vi "Get Module from Connection UI Element.vi"(10 "Alias or Full Endpoint":string, 11 "Alias Mappings by Module":T1[](array[typedef])) -> (1 "Long Endpoint":string, 2 "Short Endpoint":string, 3 "Module":string)   [LabVIEW 2020, in "Routing and Faulting System Explorer.lvlib"]
uses:
  Routing and Faulting System Explorer.lvlib
  Alias Map by Module.ctl
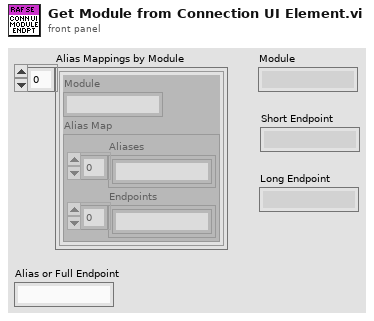
[diagram p1: front panel]
types:
  T1 = typedef "Routing and Faulting System Explorer.lvlib/Alias Map by Module.ctl" = cluster{"Module":string, "Alias Map":cluster{"Aliases":string[], "Endpoints":string[]}}
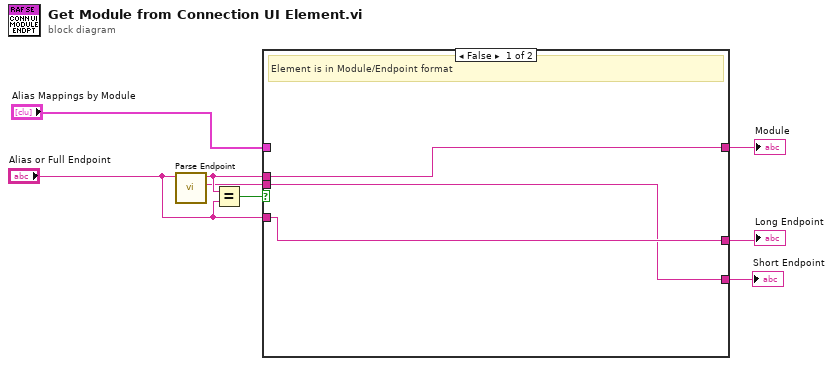
[diagram p0: block diagram]
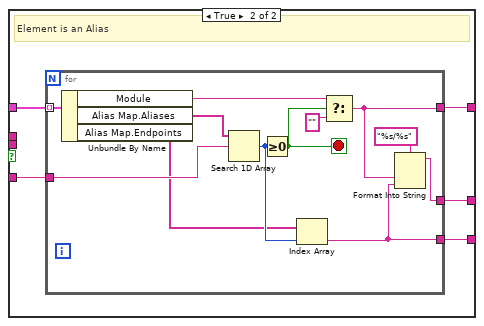
[diagram p2: hidden frame]
diagram:
  n1 = call "Parse Endpoint.vi"("Module/Endpoint"="Alias or Full Endpoint") -> ("Endpoint"=w4:string, "Module"=w6:string)  [unwired: 9 in]
  n2 = Equal?(x=w6, y="Alias or Full Endpoint") -> (x = y?=w5:bool)
  n3 = case shown="False" w5 {
    tunnel: "Alias Mappings by Module" -> [_ w16]
    tunnel: w6 -> [w11 _]
    tunnel: [w11 w15] -> w8
    tunnel: "Alias or Full Endpoint" -> [w10 w13]
    tunnel: [w9 w12] -> w1
    tunnel: w4 -> [w9 _]
    tunnel: [w10 w14] -> w2
    frame False {
      # "Element is in Module/Endpoint format"
    }
    frame True {
      # "Element is an Alias"
      n4 = for {
        tunnel: w16 -> [w28] mode=indexing
        tunnel: w13 -> [w26]
        tunnel: [w19] -> w15
        tunnel: [w18] -> w14
        tunnel: [w17] -> w12
        stop <- w25 stop-if-true
        n5 = Unbundle By Name(w28) -> ("Module"=w23:string, "Alias Map.Aliases"=w27:string[], "Alias Map.Endpoints"=w21:string[])
        n6 = Search 1D Array(1D array=w27, element=w26) -> (index of element=w22:i32)  [unwired: 1 in]
        n7 = Greater Or Equal To 0?(x=w22) -> (x >= 0?=w25:bool)
        n8 = Index Array(array=w21, index=w22) -> (element=w17:string)
        n9 = Select(t=w23, s=w25, f="") -> (s? t:f=w19:string)
        n10 = Format Into String(format string="%s/%s", w19, w17) -> (resulting string=w18:string)  [unwired: 2 in, 1 out]
      }
    }
  }
  "Module" <- w8
  "Short Endpoint" <- w1
  "Long Endpoint" <- w2
